vi "(1) Move Desired Distance (mm) - Pulse Position.vi"() -> ()   [LabVIEW 2020]
uses:
  <instrlib>/Arcus Ethernet Driver 1.0.0/ArcusEthernetComm/classes/Controller/_Controller.lvclass
panel:
  in  "Move":bool
  in  "Move X Distance (mm)":dbl
  in  "Move Y Distance (mm)":dbl
  in  "Move Z Distance (mm)":dbl
  in  "Direction Y":bool
  in  "Direcition Z":bool
  in  "Direction X":bool
  out "Scanning Rig Disconnection":errorcluster={"status"=TRUE, "code"=0, "source"=""}
  in  "error in (no error)":errorcluster
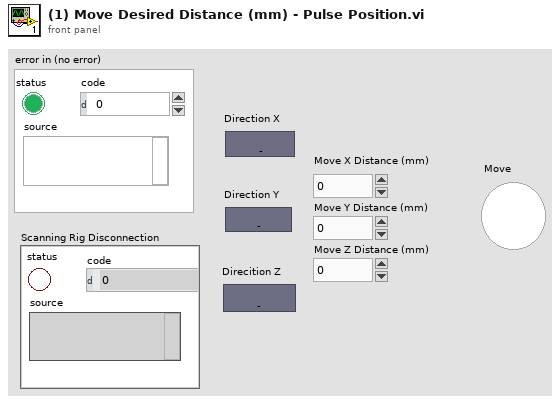
[diagram p1: front panel]
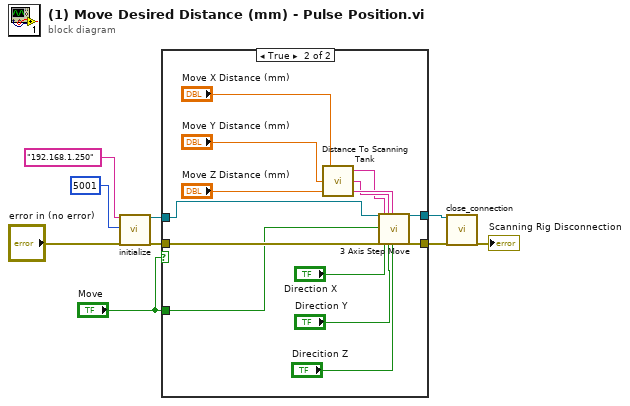
[diagram p0: block diagram]
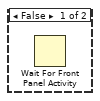
[diagram p2: hidden frame]
diagram:
  n1 = call <instrlib>:"initialize.vi"("ip_address (in)"="192.168.1.250", "dev_port(def=5001)"=u16 5001, "error in (no error)"="error in (no error)") -> ("reference (out)"=w5:refnum<class "_Controller.lvclass">, "error out"=w4:errorcluster)  [unwired: 15 in]
  n2 = case shown="True" "Move" {
    tunnel: w5 -> [_ w23]
    tunnel: w4 -> [_ w22]
    tunnel: [_ w21] -> w3
    tunnel: [_ w20] -> w2
    tunnel: "Move" -> [_ w16]
    frame False {
      n3 = Wait For Front Panel Activity() -> ()  [unwired: 3 in, 1 out]
    }
    frame True {
      n4 = call "Distance To Scanning Tank.vi"("Move Z Distance (mm)"="Move Z Distance (mm)", "Move Y Distance (mm)"="Move Y Distance (mm)", "Move X Distance (mm)"="Move X Distance (mm)") -> ("Z Steps"=w15:string, "Y Steps"=w14:string, "X Steps"=w13:string)
      n5 = call "3 Axis Step Move.vi"("reference (in)"=w23, "Move"=w16, "error in (no error)"=w22, "X Steps"=w13, "Direction X"="Direction X", "Y Steps"=w14, "Direction Y"="Direction Y", "Z Steps"=w15, "Direcition Z"="Direcition Z") -> ("reference (out)"=w21:refnum<class "_Controller.lvclass">, "error out"=w20:errorcluster)  [unwired: 17 in]
    }
  }
  n6 = call <instrlib>:"close_connection.vi"("reference (in)"=w3, "error in (no error)"=w2) -> ("error out"=→"Scanning Rig Disconnection":errorcluster)  [unwired: 16 in, 1 out]
